vi "VehicleInDistance.vi"() -> ()   [LabVIEW 2021]
uses:
  <vilib>/Instr/_visa.llb/VISA Configure Serial Port (Instr).vi
panel:
  in  "Slide":u8(slide) scale=0.0..35.0
  in  "stop":bool
  in  "VISA resource name":refnum<visa-resource-name>
  out "Waveform Chart Distance":u8(graph)
  out "Waveform Chart Error":i8(graph)
  out "Waveform Chart Load":i16(graph)
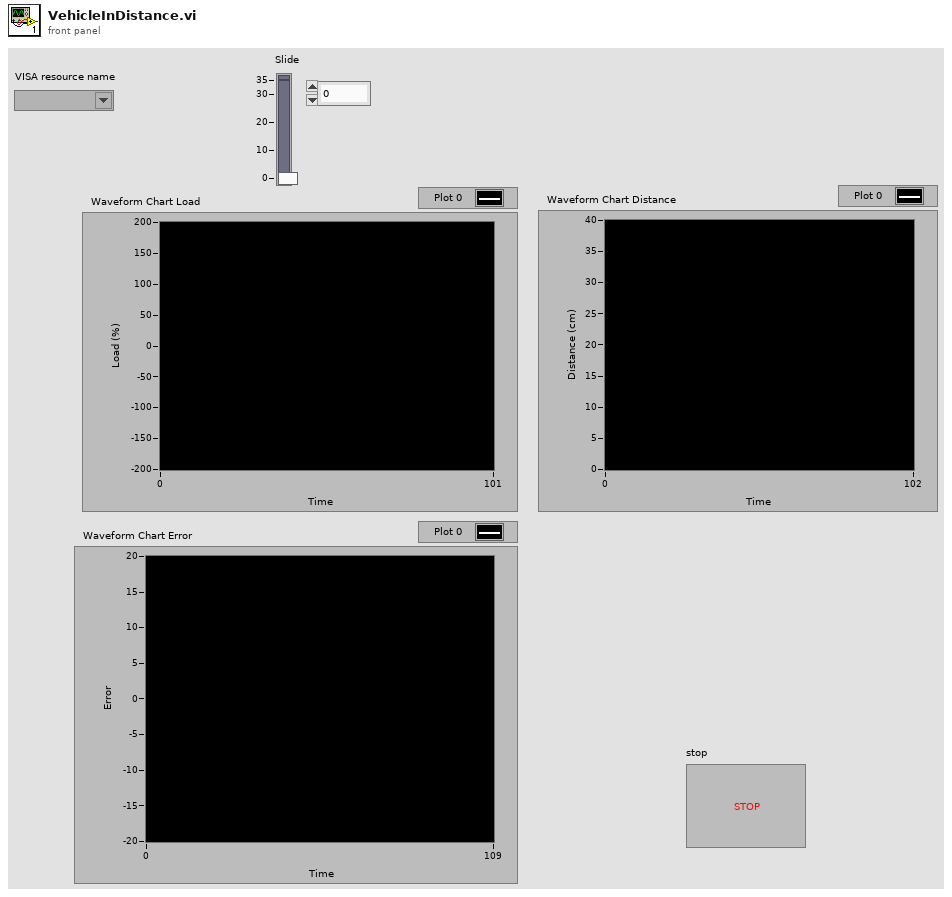
[diagram p1: front panel]
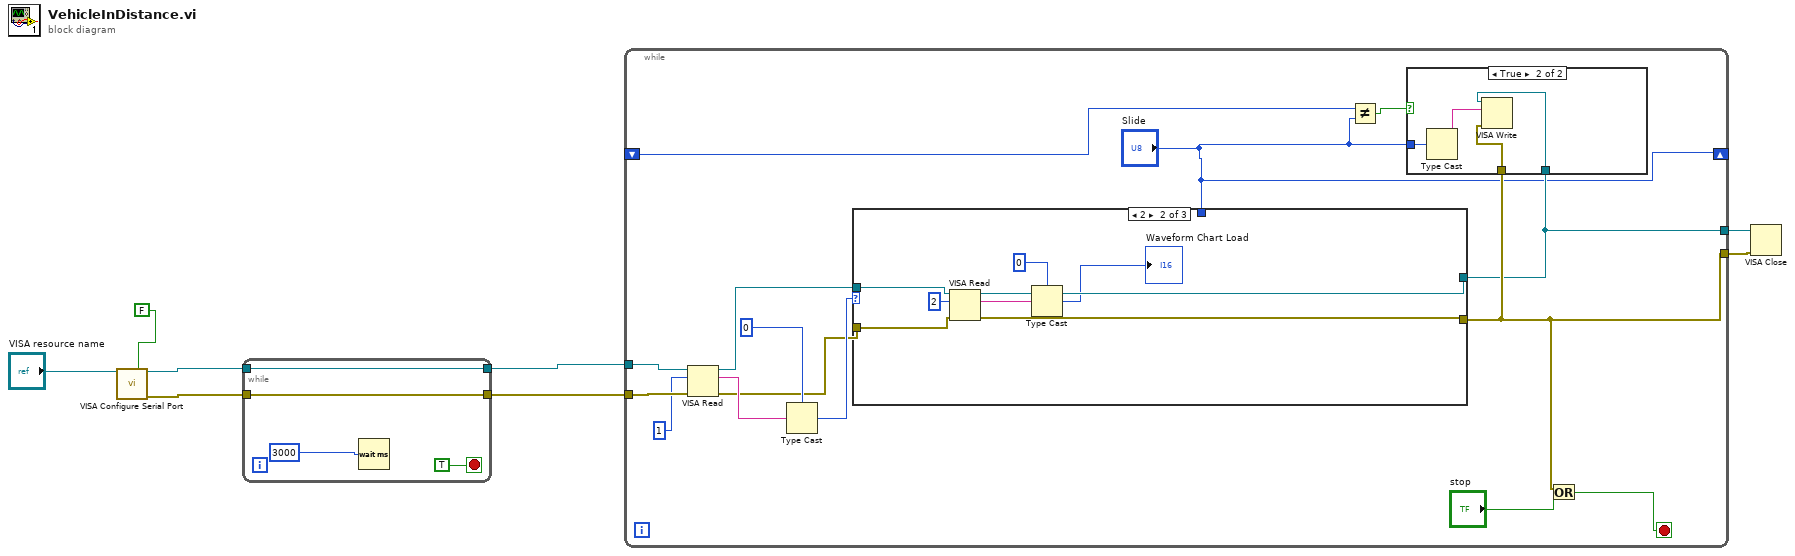
[diagram p0: block diagram]
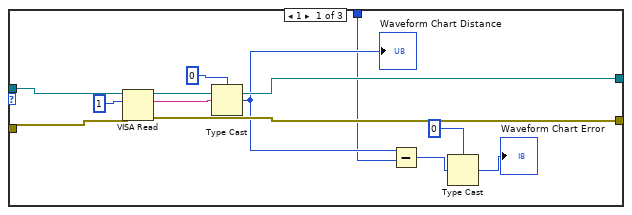
[diagram p3: hidden frame]
diagram:
  n1 = call-poly "VISA Configure Serial Port"("VISA resource name"="VISA resource name", "Enable Termination\nChar (T)"=FALSE ("Enable Termination\nChar (T)")) -> ("VISA resource name out"=w7:refnum<visa-resource-name>, "error out"=w8:errorcluster)  [unwired: 12 in]
  n2 = while {
    tunnel: w8 -> [w10]
    tunnel: w7 -> [w9]
    tunnel: [w10] -> w6
    tunnel: [w9] -> w5
    stop <- TRUE stop-if-true
    n3 = Wait (ms)(milliseconds to wait=u32 3000 ("millisecond timer value")) -> ()  [unwired: 1 out]
  }
  n4 = while {
    tunnel: w6 -> [w26]
    tunnel: w5 -> [w25]
    tunnel: [w15] -> w4
    shift-right: ["Slide"] -> _
    shift-left: _ -> [w17]
    tunnel: [w14] -> w1
    stop <- w18 stop-if-true
    n5 = VISA Read(VISA resource name=w25, byte count=u32 1, error in (no error)=w26) -> (VISA resource name out=w20:refnum<visa-resource-name>, read buffer=w23:string, error out=w21:errorcluster)  [unwired: 1 out]
    n6 = Type Cast(type=u8 0, x=w23) -> (*(type *) &x=w27:u8)
    n7 = case shown="2" w27 {
      tunnel: w20 -> [w43 w51 w53]
      tunnel: w21 -> [w42 w50 w52]
      tunnel: [w38 w46 w53] -> w14
      tunnel: [w37 w45 w52] -> w15
      tunnel: "Slide" -> [w32 _ _]
      frame 1 {
        n8 = VISA Read(VISA resource name=w43, byte count=u32 1, error in (no error)=w42) -> (VISA resource name out=w38:refnum<visa-resource-name>, read buffer=w40:string, error out=w37:errorcluster)  [unwired: 1 out]
        n9 = Type Cast(type=u8 0, x=w40) -> (*(type *) &x=w33:u8)
        "Waveform Chart Distance" <- w33
        n10 = Subtract(x=w33, y=w32) -> (x-y=w36:u8)
        n11 = Type Cast(type=i8 0, x=w36) -> (*(type *) &x=→"Waveform Chart Error":i8)
      }
      frame 2 {
        n12 = VISA Read(VISA resource name=w51, byte count=u32 2, error in (no error)=w50) -> (VISA resource name out=w46:refnum<visa-resource-name>, read buffer=w47:string, error out=w45:errorcluster)  [unwired: 1 out]
        n13 = Type Cast(type=i16 0, x=w47) -> (*(type *) &x=→"Waveform Chart Load":i16)
      }
      frame 3, Default {
      }
    }
    n14 = Not Equal?(x=w17, y="Slide") -> (x != y?=w16:bool)
    n15 = case shown="True" w16 {
      tunnel: w15 -> [_ w31]
      tunnel: w14 -> [_ w30]
      tunnel: "Slide" -> [_ w29]
      frame False {
      }
      frame True {
        n16 = Type Cast(x=w29) -> (*(type *) &x=w28:string)  [unwired: 1 in]
        n17 = VISA Write(VISA resource name=w30, write buffer=w28, error in (no error)=w31) -> ()  [unwired: 3 out]
      }
    }
    n18 = Or(x=w15, y="stop") -> (x .or. y?=w18:bool)
  }
  n19 = VISA Close(VISA resource name=w1, error in (no error)=w4) -> ()  [unwired: 1 out]
